vi "Read Type.vi"(8 "error in (no error)":errorcluster, 11 "TurnInstruction in":refnum<class "TurnInstruction.lvclass">) -> (0 "error out":errorcluster, 2 "Type":string, 3 "TurnInstruction out":refnum<class "TurnInstruction.lvclass">)   [LabVIEW 2015, in "TurnInstruction.lvclass"]
uses:
  TurnInstruction.lvclass
  Instruction.lvclass
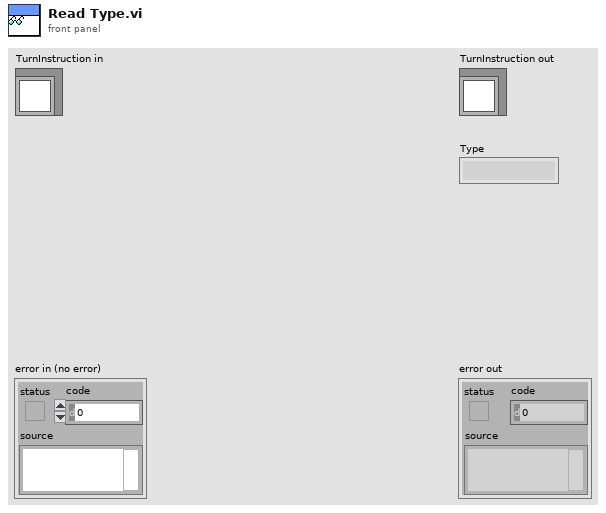
[diagram p1: front panel]
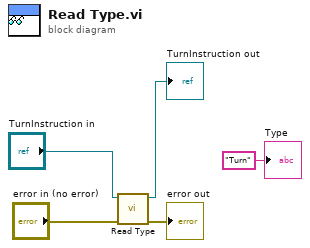
[diagram p0: block diagram]
diagram:
  n1 = call-parent "Read Type.vi"("error in (no error)"="error in (no error)", "Instruction in"="TurnInstruction in") -> ("error out"=→"error out":errorcluster, "Instruction out"=→"TurnInstruction out":refnum<class "TurnInstruction.lvclass">)  [unwired: 7 in, 1 out]
  "Type" <- "Turn" ("Type")
